vi "Untitled 5.vi"(0 "Image Src":T1, 1 "module path":path, 2 "function name":string="get_circels", 5 "session in":refnum<k35>, 7 "initialized array":dbl[][](array[numeric]), 9 "Image Dst":T1, 11 "error in (no error)":errorcluster) -> (4 "Image Out":T1, 6 "session out":refnum<k35>, 8 "BRG array":dbl[][][](array[numeric]), 13 "pellet detected?":bool, 14 "error out":errorcluster, 15 "circle info":dbl[][](array[numeric]))   [LabVIEW 2019]
uses:
  <vilib>/vision/Image Controls.llb/IMAQ Image.ctl
panel:
  out "Image":T1(plugin-control)
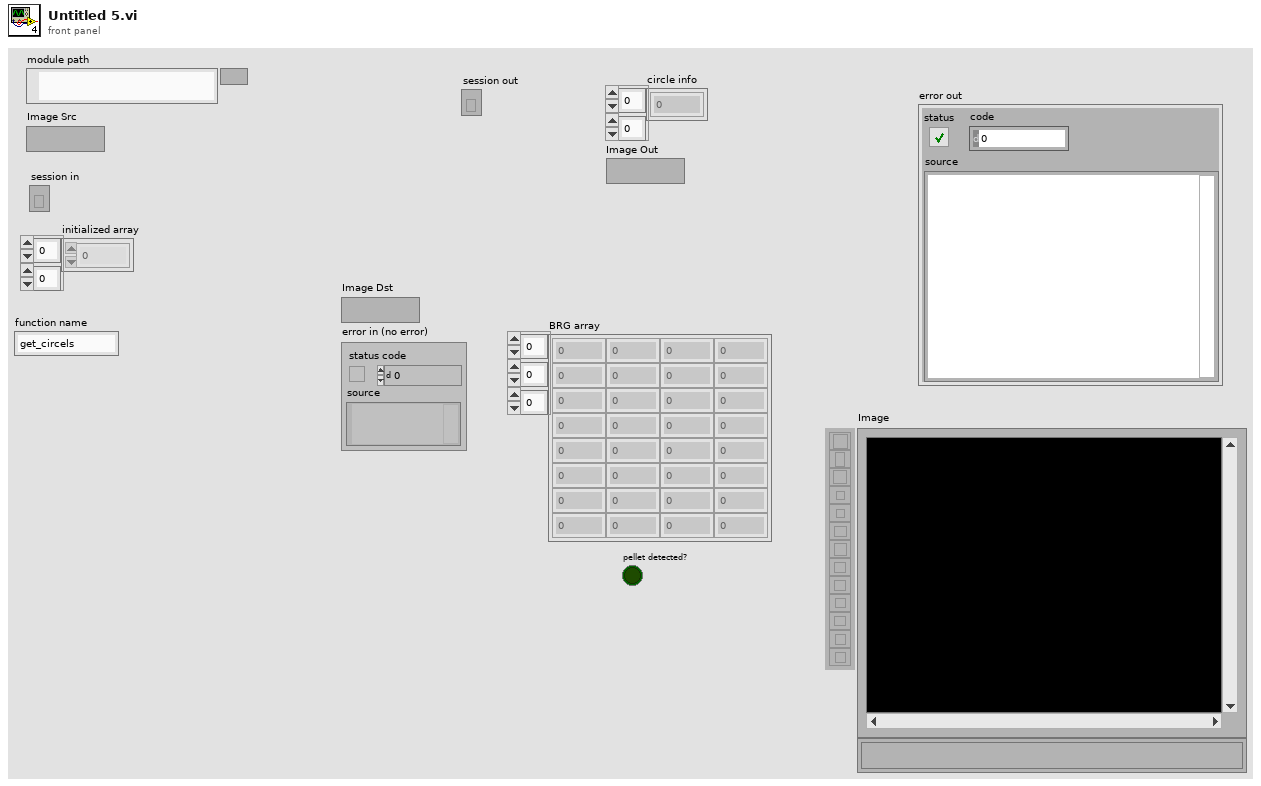
[diagram p1: front panel]
types:
  T1 = typedef "IMAQ Image.ctl" = refnum<image>
  T2 = enum32{"Invalid", "Standard", "Closed", "Hidden", "Minimized", "Maximized"}
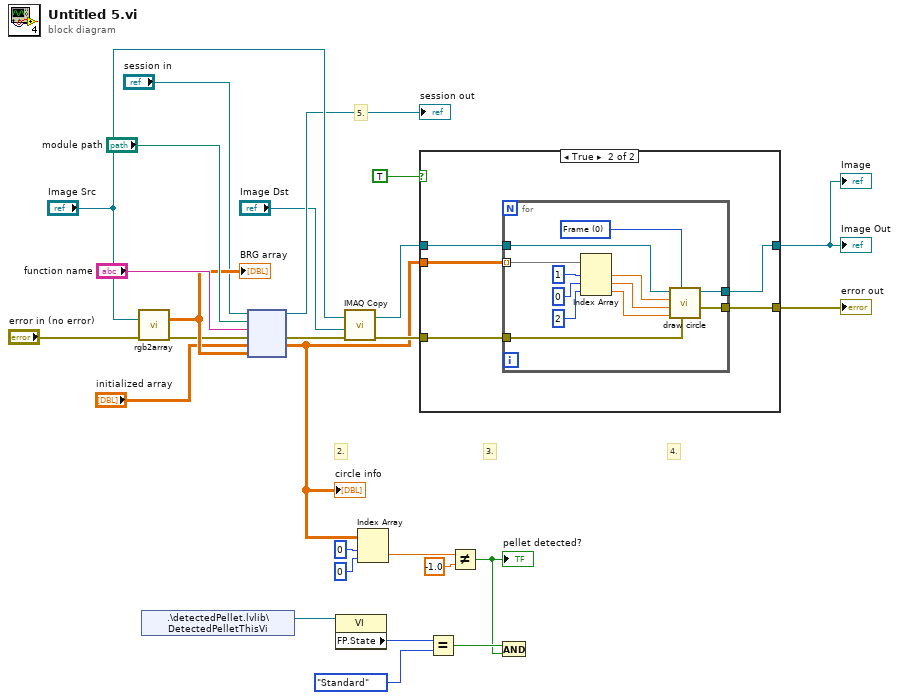
[diagram p0: block diagram]
diagram:
  # "5."
  # "4."
  # "3."
  # "2."
  n1 = call "rgb2array.vi"("Image IN"="Image Src", "error in (no error)"="error in (no error)") -> ("output Array"=w23:dbl[][][], "error out"=w15:errorcluster)  [unwired: 12 in]
  "BRG array" <- w23
  n2 = shared-variable ".\\detectedPellet.lvlib\\DetectedPelletThisVi"() -> (w12:refnum<vi>)  [unwired: 1 in, 1 out]
  n3 = node("session in", "module path", "function name", w15, "initialized array", w23) -> (→"session out":refnum<k35>, w16:errorcluster, w9:dbl[][])  [unwired: 1 in, 2 out]
  "circle info" <- w9
  n4 = property class="VI"(reference=w12) -> ("FP.State"=w11:T2)  [unwired: 1 in, 2 out]
  n5 = call "IMAQ Copy"("error in (no error)"=w16, "Image Dst"="Image Dst", "Image Src"="Image Src") -> ("error out"=w24:errorcluster, "Image Dst Out"=w13:T1)  [unwired: 3 in]
  n6 = Index Array(array=w9, index (row)=0, index (col)=0 ("disabled index (col)")) -> (element=w6:dbl)
  n7 = case shown="True" TRUE {
    tunnel: w24 -> [w27 w33]
    tunnel: w9 -> [_ w32]
    tunnel: [w27 w31] -> w19
    tunnel: w13 -> [w28 w30]
    tunnel: [w28 w29] -> w1
    frame False {
    }
    frame True {
      n8 = for {
        tunnel: w30 -> [w45]
        tunnel: w32 -> [w44] mode=indexing
        tunnel: w33 -> [w36]
        tunnel: [w35] -> w31
        tunnel: [w34] -> w29
        w37 = u32 0 items=["Frame", "Fill"] ("Drawing Mode (Frame)")
        n9 = Index Array(array=w44, index #1=1 ("index"), index #2=0 ("index"), index #3=2 ("index")) -> (element #1=w40:dbl, element #2=w39:dbl, element #3=w38:dbl)
        n10 = call "draw circle.vi"("error in (no error)"=w36, "Drawing Mode (Frame)"=w37, "box size"=w38, "Y"=w39, "X"=w40, "Image In"=w45) -> ("error out"=w35:errorcluster, "Image Out"=w34:T1)  [unwired: 4 in]
      }
    }
  }
  "Image Out" <- w1
  "error out" <- w19
  "Image" <- w1
  n11 = Equal?(x=w11, y=T2."Standard") -> (x = y?=w4:bool)
  n12 = Not Equal?(x=w6, y=-1.0) -> (x != y?=w3:bool)
  "pellet detected?" <- w3
  n13 = And(x=w4, y=w3) -> ()  [unwired: 1 out]
